vi "Handle Tree Run Time Menu Item Select.vi"(6 "Coords":T1, 8 "error in (no error)":errorcluster, 9 "ItemPath":string, 10 "ItemTag":string, 11 "Process Explorer View in":refnum<class "Process Explorer View.lvclass">) -> (0 "error out":errorcluster, 3 "Process Explorer View out":refnum<class "Process Explorer View.lvclass">)   [LabVIEW 2019, in "Process Explorer View.lvclass"]
doc: "<RequiredOverrideReason>The action to take for a given Right-click run time menu selection in the file explorer tree.</RequiredOverrideReason>"
uses:
  <vilib>/gpm_packages/@cs/Car-wash/Source/Process Explorer View/Process Explorer View.lvclass
  C:/Program Files/National Instruments/LabVIEW 2019/vi.lib/gpm_packages/@cs/file-explorer-extension/Source/File Explorer/File Explorer/File Explorer.lvclass
  <vilib>/Utility/miscctls.llb/LVPoint32TypeDef.ctl
  <vilib>/gpm_packages/@cs/file-explorer-extension/Source/File Explorer/File Explorer/File Explorer.lvclass/File Explorer.ctl
  <vilib>/gpm_packages/@cs/Test-executive-builder/Source/Application Dependencies/Create Test Executive.ctl
  <vilib>/gpm_packages/@cs/file-explorer-extension/Source/File Explorer/File Explorer/File Explorer.lvclass
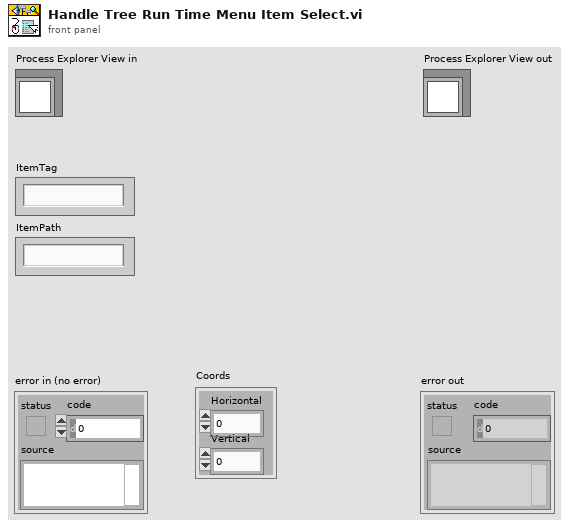
[diagram p1: front panel]
types:
  T1 = typedef "LVPoint32TypeDef.ctl" = cluster{"Horizontal":i32, "Vertical":i32}
  T2 = typedef "Create Test Executive.ctl" = cluster{"Folder Path":path, "File Name with Extension":string}
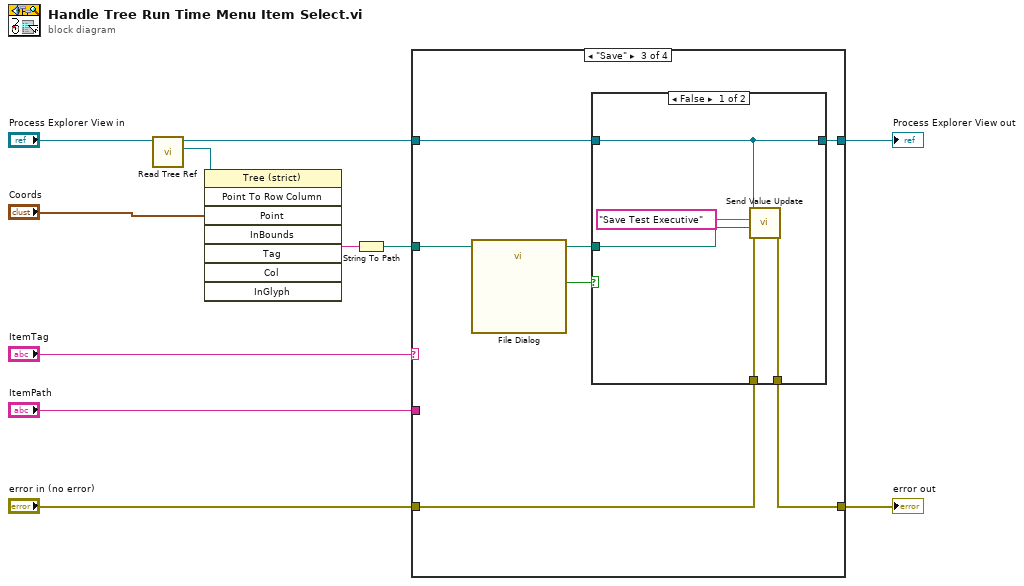
[diagram p0: block diagram]
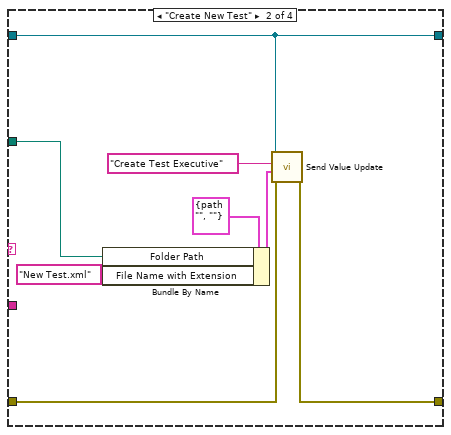
[diagram p3: hidden frame]
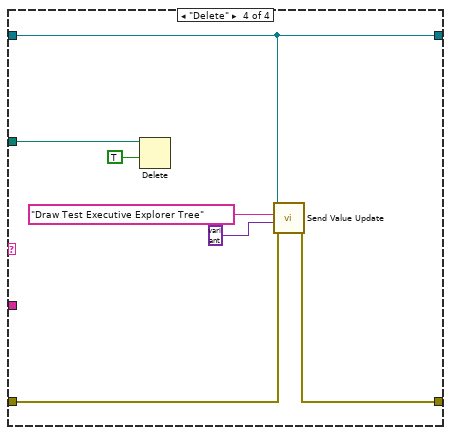
[diagram p5: hidden frame]
diagram:
  n1 = call <vilib>:"Read Tree Ref.vi"("File Explorer in"="Process Explorer View in") -> ("Tree Ref"=w11:refnum<vi>, "File Explorer out"=w10:refnum<class "Process Explorer View.lvclass">)  [unwired: 8 in, 1 out]
  n2 = invoke class="Tree (strict)" method="Point To Row Column"(reference=w11, "Point"="Coords") -> ("Tag"=w9:string)  [unwired: 6 in, 7 out]
  n3 = String To Path(string=w9) -> (path=w8:path)
  n4 = case shown="\"Save\"" "ItemTag" {
    tunnel: "ItemPath" -> [_ _ _ _]
    tunnel: [w13 w21 w23 w40] -> w6
    tunnel: w10 -> [w13 w21 w28 w40]
    tunnel: [w12 w18 w26 w36] -> w1
    tunnel: "error in (no error)" -> [w12 w19 w27 w37]
    tunnel: w8 -> [_ w15 w25 w42]
    frame Default {
    }
    frame "Create New Test" {
      n5 = Bundle By Name(cluster=T2 {"Folder Path"=path "", "File Name with Extension"=""} ("Create Test Executive"), "Folder Path"=w15, "File Name with Extension"="New Test.xml") -> (w16:T2)
      n6 = call-dynamic "Send Value Update.vi"("error in (no error)"=w19, "Value"=w16, "Datum Name"="Create Test Executive", "IViewable in"=w21) -> ("error out"=w18:errorcluster)  [unwired: 7 in]
    }
    frame "Save" {
      n7 = call "File Dialog"("start path"=w25) -> ("selected path"=w24:path, "cancelled"=w22:bool)  [unwired: 11 in, 2 out]
      n8 = case shown="False" w22 {
        tunnel: w28 -> [w29 w35]
        tunnel: w27 -> [w32 w34]
        tunnel: [w31 w34] -> w26
        tunnel: w24 -> [w30 _]
        tunnel: [w29 w35] -> w23
        frame False {
          n9 = call-dynamic "Send Value Update.vi"("error in (no error)"=w32, "Value"=w30, "Datum Name"="Save Test Executive", "IViewable in"=w29) -> ("error out"=w31:errorcluster)  [unwired: 7 in]
        }
        frame True {
        }
      }
    }
    frame "Delete" {
      n10 = Delete(path (use dialog)=w42, confirm (F)=TRUE) -> ()  [unwired: 3 in, 3 out]
      n11 = call-dynamic "Send Value Update.vi"("error in (no error)"=w37, "Value"=variant ("Data Type"), "Datum Name"="Draw Test Executive Explorer Tree", "IViewable in"=w40) -> ("error out"=w36:errorcluster)  [unwired: 7 in]
    }
  }
  "error out" <- w1
  "Process Explorer View out" <- w6
